vi "warning display.vi"(9 "TempD(K) 2":dbl, 10 "TempB(K) 2":dbl, 11 "Field(Oe) 2":dbl) -> ()   [LabVIEW 2019]
panel:
  out "TempD(K)":dbl
  out "TempB(K)":dbl
  out "Field(Oe)":dbl
  out "Field ON":bool
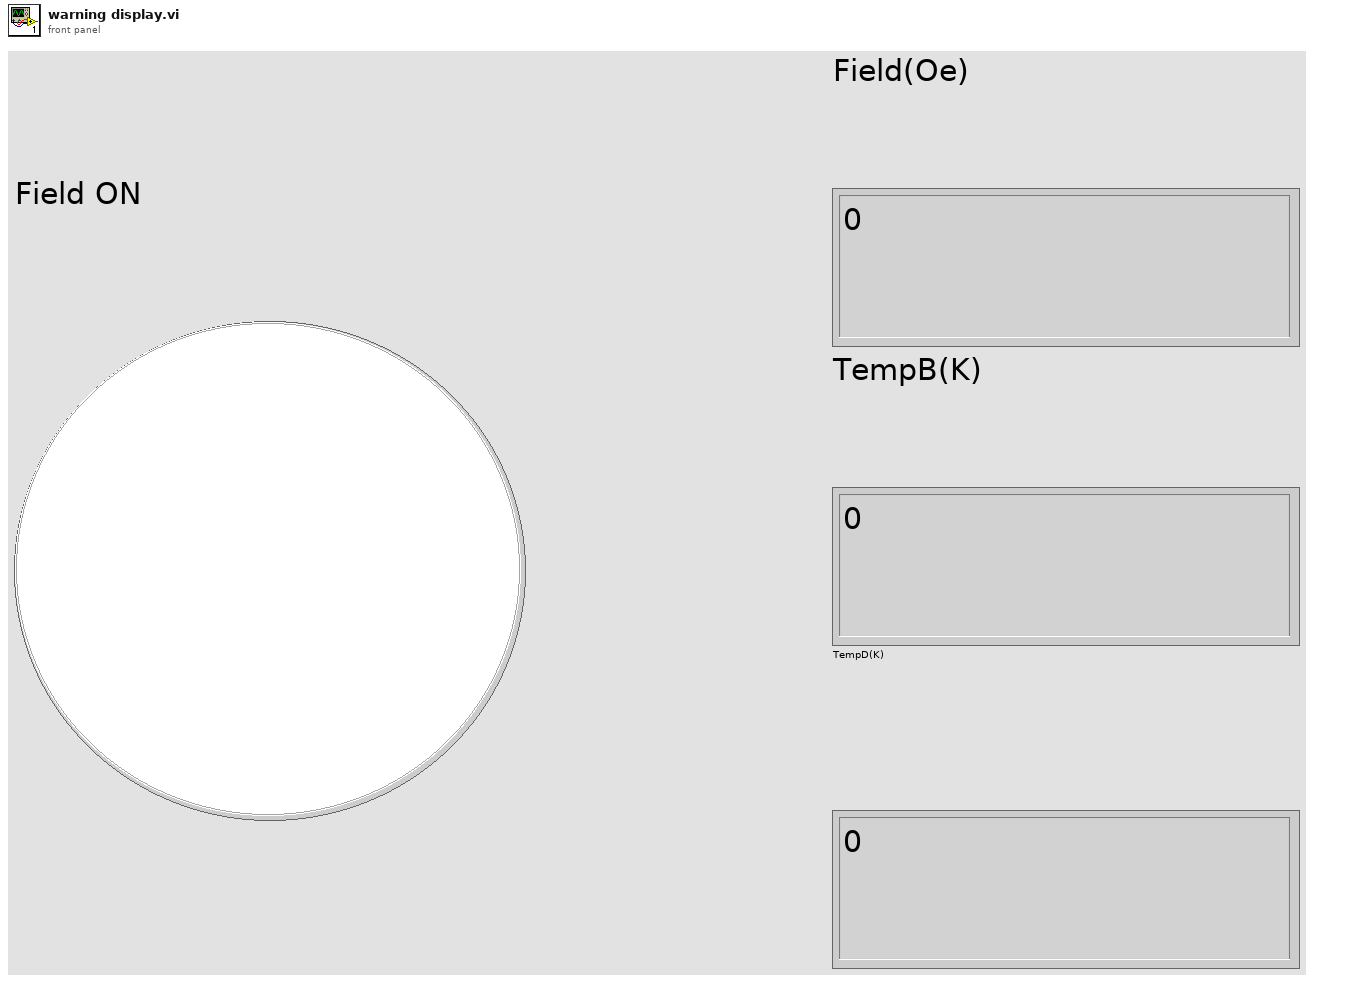
[diagram p1: front panel]
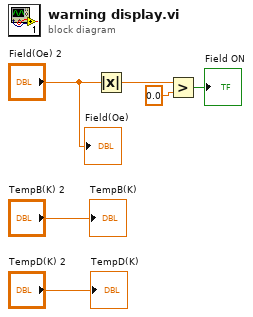
[diagram p0: block diagram]
diagram:
  n1 = Absolute Value(x="Field(Oe) 2") -> (abs(x)=w3:dbl)
  n2 = Greater?(x=w3, y=0.0) -> (0:→"Field ON":bool)
  "Field(Oe)" <- "Field(Oe) 2"
  "TempB(K)" <- "TempB(K) 2"
  "TempD(K)" <- "TempD(K) 2"
